vi "Read XML.vi"(8 "error in (no error)":errorcluster, 11 "Configuration in":refnum<class "Configuration.lvclass">) -> (0 "error out":errorcluster, 2 "XML Elements":string[](array[string]), 3 "Configuration out":refnum<class "Configuration.lvclass">)   [LabVIEW 2011, in "Configuration.lvclass"]
uses:
  Configuration.lvclass
  Configuration.lvclass/Configuration.ctl
  <vilib>/Utility/xml.llb/Read From XML File(array).vi
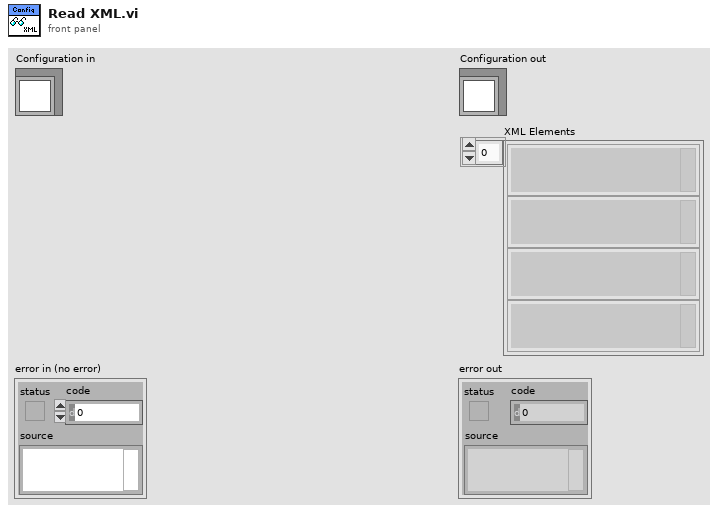
[diagram p1: front panel]
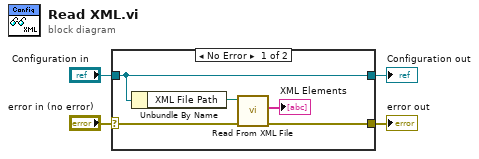
[diagram p0: block diagram]
diagram:
  n1 = case shown="No Error" "error in (no error)" {
    selector: "error in (no error)" -> [w7 w11]
    tunnel: [w6 w11] -> w3
    tunnel: [w9 w10] -> w1
    tunnel: "Configuration in" -> [w9 w10]
    frame No Error {
      n2 = Unbundle By Name(w9) -> ("XML File Path"=w8:path)
      n3 = call-poly <vilib>:"Read From XML File.vi"("error in (no error)"=w7, "XML File Path"=w8) -> ("error out"=w6:errorcluster, "XML Elements"=→"XML Elements":string[])  [unwired: 7 in, 1 out]
    }
    frame Error {
    }
  }
  "error out" <- w3
  "Configuration out" <- w1
